vi "Update Process Indicator.vi"(8 "error in (no error)":errorcluster, 11 "Tamer in":refnum<class "Tamer.lvclass">) -> (0 "error out":errorcluster, 3 "Tamer out":refnum<class "Tamer.lvclass">)   [LabVIEW 2020, in "Tamer.lvlib" / "Tamer.lvclass"]
uses:
  Tamer.lvclass
  C:/Users/marco/Documents/GitHub_Lab/TALOS/talos/Father of all uServices/Father of all uServices/Father of all uServices.lvclass
  Tamer.lvclass/Tamer.ctl
  Ancestor/Ancestor/Ancestor.lvclass/Ancestor.ctl
  Support VIs/Generate Error.vi
  FGV/Error Memory/Get Error Description.vi
  Support VIs/Get PC name.vi
  Ancestor/Ancestor/Read ID.vi
  Support VIs/Get Class Name.vi
  <vilib>/Utility/error.llb/Clear Errors.vi
  FGV/Error Memory/Error Memory Core.vi
  <vilib>/AdvancedString/Delimited String to 1D String Array.vi
  Support VIs/Circus Root Path.vi
  FGV/Error Memory/Error Crt Lvl checker.vi
  FGV/Error Memory/Error Memory Core.vi/40c8088d-b597-4017-91af-faa98e00292e.vi
  FGV/Error Memory/Error Memory Core.vi/d4a3ab98-063c-4e44-b43d-fbdcfe6c2be2.vi
  Support VIs/Global Memory.vi
  <vilib>/Utility/LVClass/Get LV Class Name.vi
  Support VIs/Is in Packed Library.vi
  Support VIs/TALOS Root path.vi
  Support VIs/Read CSV worksheet.vi
  Support VIs/Global Constants.vi
  <vilib>/Utility/error.llb/General Error Handler.vi
  Support VIs/Error Log.vi
  Ancestor/Ancestor/Ancestor.lvclass
  <vilib>/Comparison/Equal/Equal Functor/Equal Functor.lvclass
  Father of all uServices/Father of all uServices/Father of all uServices.lvclass
  TALOS.lvlib
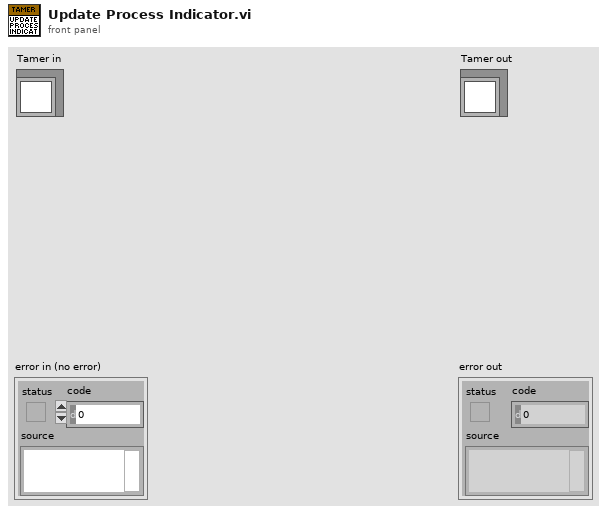
[diagram p1: front panel]
types:
  T1 = cluster{"delimited string":string, "Process ID":string}
  T2 = cluster{"delimited string":string, "Process ID":string}[]
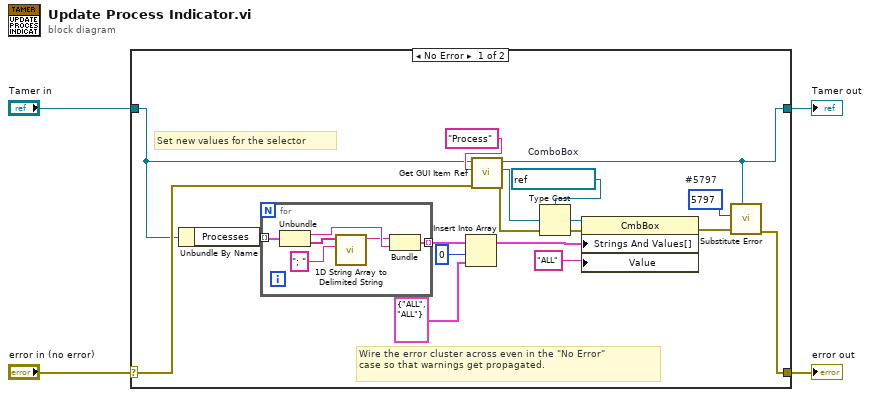
[diagram p0: block diagram]
diagram:
  n1 = case shown="No Error" "error in (no error)" {
    selector: "error in (no error)" -> [w21 w29]
    tunnel: [w8 w29] -> w3
    tunnel: [w7 w28] -> w1
    tunnel: "Tamer in" -> [w11 w28]
    frame No Error {
      w6 = 5797  # #5797
      w13 = refnum<vi> refnum  # ComboBox
      # "Set new values for the selector"
      # "Wire the error cluster across even in the \"No Error\"\ncase so that warnings get propagated."
      n2 = Unbundle By Name(w11) -> ("Processes"=w17:map{string, string[]})
      n3 = for {
        tunnel: w17 -> [w26] mode=indexing
        tunnel: [w27] -> w20 mode=indexing
        n4 = Unbundle(w26) -> ("Process ID"=w23:string, "Monkeys"=w25:string[])
        n5 = call <vilib>:"1D String Array to Delimited String.vi"("delimiter"="; " ("Separator"), "string array"=w25) -> ("delimited string"=w22:string)  [unwired: 9 in]
        n6 = Bundle("delimited string"=w22, "Process ID"=w23) -> (w27:T1)  [unwired: 1 in]
      }
      n7 = Insert Into Array(array=w20, index=0, new element=cluster{"Process ID":string, string} {"Process ID"="ALL", "ALL"} ("new element/subarray")) -> (w19:T2)
      n8 = call "Get GUI Item Ref.vi"("error in (no error)"=w21, "FP Item Name"="Process", "uService Template in"=w11) -> ("error out"=w18:errorcluster, "Ctl Refnum"=w16:refnum<vi>, "uService Template out"=w7:refnum<class "Tamer.lvclass">)  [unwired: 6 in]
      n9 = Type Cast(type=w13, x=w16) -> (*(type *) &x=w15:refnum<vi>)
      n10 = property class="CmbBox"(reference=w15, error in=w18, "Strings And Values[]"=w19, "Value"="ALL") -> (error out=w9:errorcluster)  [unwired: 1 out]
      n11 = call "Substitute Error.vi"("LabVIEW Object"=w7, "error in (no error)"=w9, "Error Code"=w6) -> ("error out"=w8:errorcluster)  [unwired: 8 in]
    }
    frame Error {
    }
  }
  "error out" <- w3
  "Tamer out" <- w1
